vi "TAT-PLC Alarm Data.vi"(8 "error in (no error)":errorcluster, 11 "Modbus instance in":refnum<class "Modbus API.lvclass">) -> (0 "error out":errorcluster, 1 "Alarm Enable-2":bool, 2 "T - Alarm":u16[](array[numeric]), 3 "Modbus instance out":refnum<class "Modbus API.lvclass">, 5 "Alarm Enable-1":bool, 7 "Ass Alarm":u16[](array[numeric]))   [LabVIEW 2017]
uses:
  <vilib>/NI/Modbus Library/API/Modbus API.lvclass
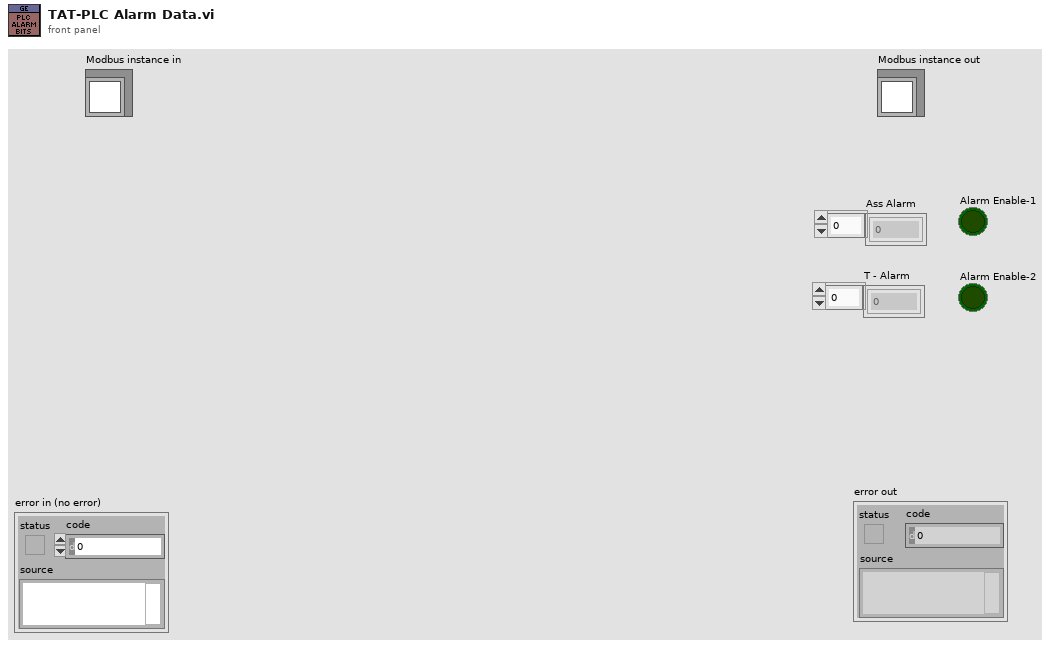
[diagram p1: front panel]
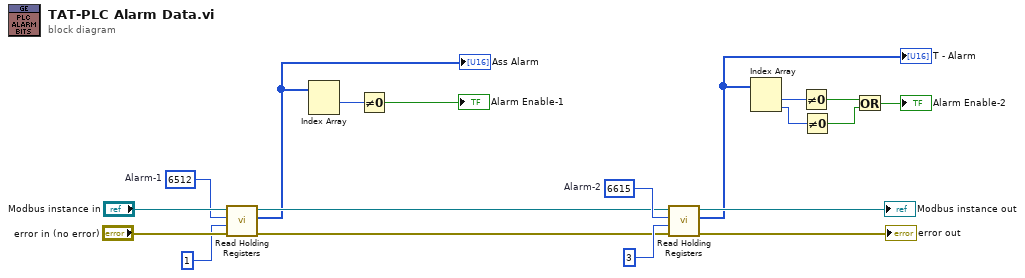
[diagram p0: block diagram]
diagram:
  w9 = u16 6615  # Alarm-2
  w15 = u16 6512  # Alarm-1
  n1 = call-dynamic "Read Holding Registers.vi"("error in"="error in (no error)", "number of inputs"=u16 1, "starting address"=w15, "Modbus instance in"="Modbus instance in") -> ("error out"=w4:errorcluster, "register values"=w2:u16[], "Modbus instance out"=w6:refnum<class "Modbus API.lvclass">)  [unwired: 5 in]
  "Ass Alarm" <- w2
  n2 = Index Array(array=w2) -> (element #1=w18:u16)  [unwired: 2 in, 1 out]
  n3 = Not Equal To 0?(x=w18) -> (x != 0?=→"Alarm Enable-1":bool)
  n4 = call-dynamic "Read Holding Registers.vi"("error in"=w4, "number of inputs"=u16 3, "starting address"=w9, "Modbus instance in"=w6) -> ("error out"=→"error out":errorcluster, "register values"=w1:u16[], "Modbus instance out"=→"Modbus instance out":refnum<class "Modbus API.lvclass">)  [unwired: 5 in]
  "T - Alarm" <- w1
  n5 = Index Array(array=w1) -> (element #1=w8:u16, element #2=w11:u16)  [unwired: 2 in]
  n6 = Not Equal To 0?(x=w8) -> (x != 0?=w7:bool)
  n7 = Not Equal To 0?(x=w11) -> (x != 0?=w13:bool)
  n8 = Or(x=w7, y=w13) -> (x .or. y?=→"Alarm Enable-2":bool)
